vi "Load Config.vi"(8 "error in (no error)":errorcluster, 11 "System Health Module in":refnum<class "System Health Module.lvclass">) -> (0 "error out":errorcluster, 3 "System Health Module out":refnum<class "System Health Module.lvclass">)   [LabVIEW 2020, in "Volatus.lvlib" / "System Health Module.lvclass"]
uses:
  System Health Module.lvclass
  C:/dev/lv20CE/relink/lv-volatus/Volatus/Module/Module.lvclass
  Module/Module.lvclass/Module.ctl
  VolatusConfig/VolatusConfigElement/VolatusConfigElement.lvclass/VolatusConfigElement.ctl
  Drive Info.ctl
  Drive Config.ctl
  System Health Module.lvclass/System Health Module.ctl
  Module/Config.vi
  VolatusConfig/VolatusConfigElement/Element.vi
  VolatusConfig/Task/Task Config.lvclass
  C:/dev/lv20CE/relink/lv-volatus/VolatusConfig/VolatusConfigElement/VolatusConfigElement.lvclass
  VolatusConfig/Group/Group Config.lvclass
  Module/Module.lvclass
  VolatusConfig/VolatusConfigElement/VolatusConfigElement.lvclass
  lv-cdm/CDM-Config/Config Element/Config Element.lvclass
  C:/dev/lv20CE/relink/lv-volatus/Volatus/System Health Module/System Health Module.lvclass
  C:/dev/lv20CE/relink/lv-volatus/VolatusConfig/Task/Task Config.lvclass
  C:/dev/lv20CE/relink/lv-volatus/VolatusConfig/Group/Group Config.lvclass
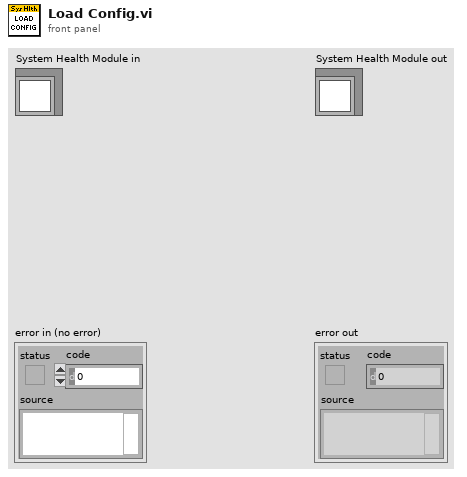
[diagram p1: front panel]
types:
  T1 = typedef "Volatus.lvlib/System Health Module.lvclass/Drive Info.ctl" = cluster{"Config":T2, "Capacity GB":dbl, "Used GB":dbl, "Next Warning":dbl, "Next Error":dbl}
  T2 = typedef "Volatus.lvlib/System Health Module.lvclass/Drive Config.ctl" = cluster{"Path":path, "Warning GB":dbl, "Error GB":dbl}
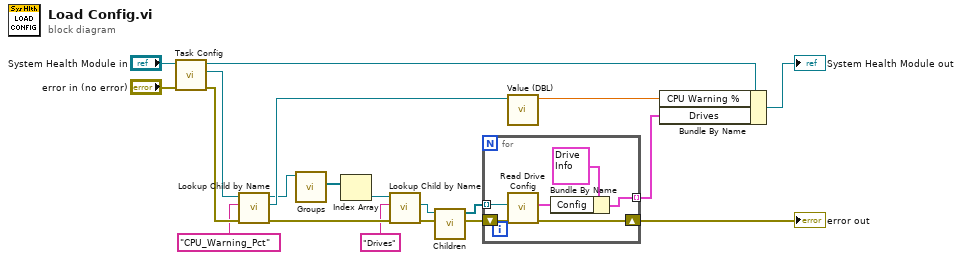
[diagram p0: block diagram]
diagram:
  n1 = call "Task Config.vi"("error in (no error)"="error in (no error)", "Module in"="System Health Module in") -> ("error out"=w19:errorcluster, "Task Config"=w7:refnum<class "Task Config.lvclass">, "Module out"=w16:refnum<class "System Health Module.lvclass">)  [unwired: 7 in]
  n2 = call "Lookup Child by Name.vi"("error in (no error)"=w19, "Child Name"="CPU_Warning_Pct", "VolatusConfigElement in"=w7) -> ("error out"=w20:errorcluster, "Child"=w5:refnum<class "Config Element.lvclass">, "VolatusConfigElement out"=w2:refnum<class "Task Config.lvclass">)  [unwired: 5 in, 1 out]
  n3 = call "Groups.vi"("Task in"=w2) -> ("Groups"=w3:refnum<class "Group Config.lvclass">[])  [unwired: 8 in, 2 out]
  n4 = Index Array(array=w3) -> (element=w1:refnum<class "Group Config.lvclass">)  [unwired: 1 in]
  n5 = call "Lookup Child by Name.vi"("error in (no error)"=w20, "Child Name"="Drives", "VolatusConfigElement in"=w1) -> ("error out"=w14:errorcluster, "Child"=w13:refnum<class "Config Element.lvclass">)  [unwired: 5 in, 2 out]
  n6 = call "Children.vi"("error in (no error)"=w14, "Config Element in"=w13) -> ("error out"=w12:errorcluster, "Elements"=w11:refnum<class "Config Element.lvclass">[])  [unwired: 8 in]
  n7 = for {
    tunnel: w11 -> [w25] mode=indexing
    shift-right: [w22] -> w8
    shift-left: w12 -> [w26]
    tunnel: [w21] -> w9 mode=indexing
    n8 = call "Read Drive Config.vi"("error in (no error)"=w26, "Drive Config Element"=w25) -> ("error out"=w22:errorcluster, "Drive Config"=w23:T2)  [unwired: 8 in]
    n9 = Bundle By Name(cluster=T1 {"Config"={"Path"=path "", "Warning GB"=0.0, "Error GB"=0.0}, "Capacity GB"=0.0, "Used GB"=0.0, "Next Warning"=0.0, "Next Error"=0.0} ("Drive Info"), "Config"=w23) -> (w21:T1)
  }
  "error out" <- w8
  n10 = call "Value (DBL).vi"("Config Element in"=w5) -> ("DBL Value"=w4:dbl)  [unwired: 9 in, 1 out]
  n11 = Bundle By Name(cluster=w16, "CPU Warning %"=w4, "Drives"=w9) -> (→"System Health Module out":refnum<class "System Health Module.lvclass">)
